vi "CALC_MARK_FUNC_APE_THR.vi"(0 "VISA IN":refnum<visa-resource-name>, 1 "Marker number":i32, 2 "Threshold Value":i32, 5 "error in":errorcluster, 7 "Channel":i32) -> (14 "VISA Out":refnum<visa-resource-name>, 19 "error out":errorcluster)   [LabVIEW 2018, in "PNA-X.lvlib"]
doc: "CALCulate<cnum>:MARKer<mkr>:FUNCtion:APEak:THReshold <num> \n(Read-Write) Sets peak threshold for the specified marker. If a peak (using the criteria set with \n:EXCursion) is below this reference value, it will not be considered when searching for peaks. This \ncommand applies to marker peak searches (Next peak, Peak Right, Peak Left). \nSee Critical Note \nParameters \n<cnum> Channel number of the measurement. There must be a selected measurement \non that channel. If unspecified, <cnum> is set to 1. \n<mkr> Any marker number from 1 to 10; if unspecified, value is set to 1 \n<num> Threshold value.Choose any number between -500 and 500. \nNote: This command will accept MIN or MAX instead of a numeric \nparameter. See SCPI Syntax for more information. \nExamples CALC:MARK:FUNC:APE:THR -40 \ncalculate2:marker8:function:apeak:threshold -55 \n1533\n\nQuery Syntax CALCulate<cnum>:MARKer<mkr>:FUNCtion:APEak:THReshold? \nReturn Type Numeric \nDefault -100"
uses:
  PNA-X.lvlib
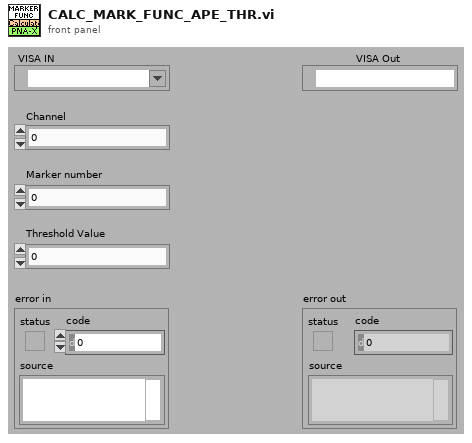
[diagram p1: front panel]
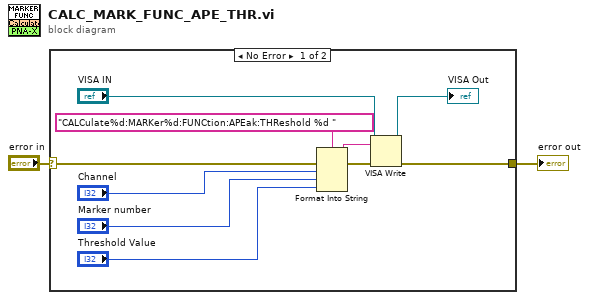
[diagram p0: block diagram]
diagram:
  n1 = case shown="No Error" "error in" {
    selector: "error in" -> [w12 w13]
    tunnel: [w7 w13] -> w1
    frame No Error {
      n2 = Format Into String(format string="CALCulate%d:MARKer%d:FUNCtion:APEak:THReshold %d " ("Cmdline"), error in=w12, "Channel", "Marker number", "Threshold Value") -> (resulting string=w10:string, error out=w11:errorcluster)  [unwired: 1 in]
      n3 = VISA Write(VISA resource name="VISA IN", write buffer=w10, error in (no error)=w11) -> (VISA resource name out=→"VISA Out":refnum<visa-resource-name>, error out=w7:errorcluster)  [unwired: 1 out]
    }
    frame Error {
    }
  }
  "error out" <- w1
